vi "Clear.vi"(3 "输入":u32[][](array[numeric])) -> (0 "清除行":i16[](array[numeric]), 1 "得分":dbl)   [LabVIEW 2016]
panel:
  out "清除":bool
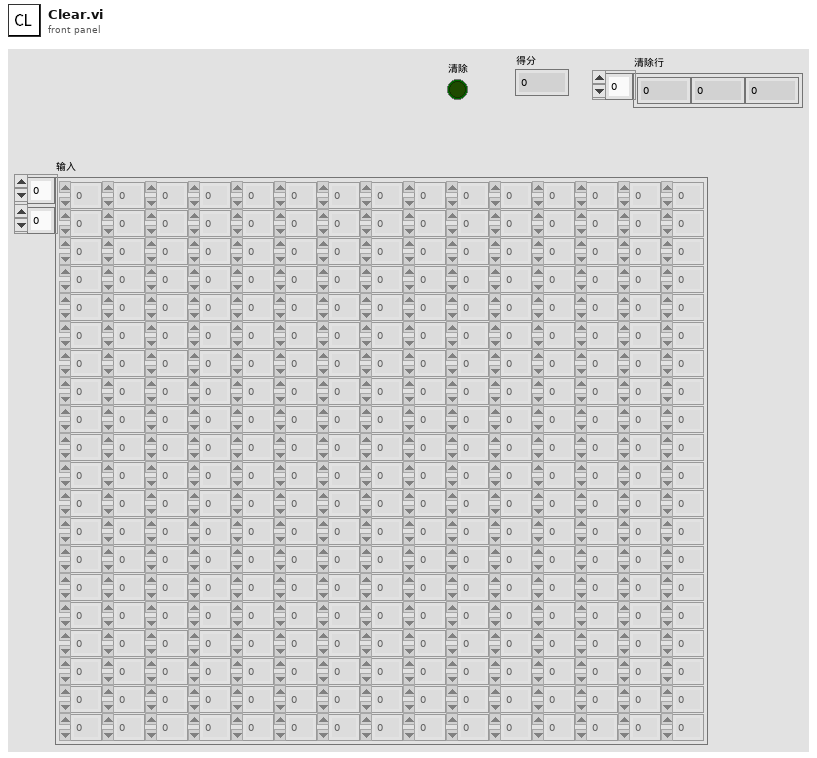
[diagram p1: front panel]
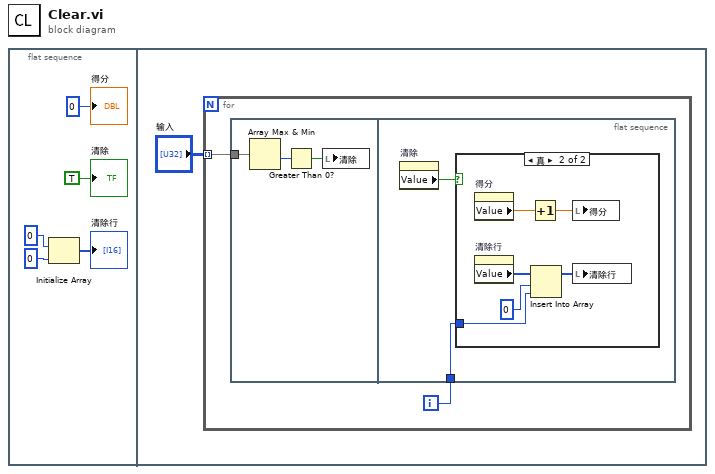
[diagram p0: block diagram]
diagram:
  n1 = flat-sequence {
    frame #0 {
      n2 = Initialize Array(0, 0) -> (→"清除行":i32[])
      "得分" <- 0
      "清除" <- TRUE
    }
    frame #1 {
      n3 = for {
        tunnel: "输入" -> [w8] mode=indexing
        i -> [w7]
        n4 = flat-sequence {
          tunnel: w8 -> [w11]
          tunnel: w7 -> [w12]
          frame #0 {
            n5 = Array Max & Min(array=w11) -> (min value=w10:u32)  [unwired: 3 out]
            n6 = Greater Than 0?(x=w10) -> (x > 0?=w9:bool)
            n7 = local write "清除"(w9) -> ()
          }
          frame #1 {
            n8 = property on="清除" class="Bool (严格)"() -> ("Value"=w13:bool)  [unwired: 2 in, 2 out]
            n9 = case shown="真" w13 {
              tunnel: w12 -> [_ w17]
              frame False {
              }
              frame True {
                n10 = property on="得分" class="DigNum (严格)"() -> ("Value"=w15:dbl)  [unwired: 2 in, 2 out]
                n11 = property on="清除行" class="Arr (严格)"() -> ("Value"=w19:i16[])  [unwired: 2 in, 2 out]
                n12 = Increment(x=w15) -> (x+1=w14:dbl)
                n13 = Insert Into Array(array=w19, index=0, new element=w17) -> (w18:i16[])
                n14 = local write "得分"(w14) -> ()
                n15 = local write "清除行"(w18) -> ()
              }
            }
          }
        }
      }
    }
  }
